vi "Z Aux Direct Move Smooth.vi"(0 "handle":u32, 1 "next1":sgl, 2 "next3":sgl, 5 "end1":sgl, 7 "end2":sgl, 9 "end3":sgl, 11 "error in (no error)":errorcluster caption="错误输入（无错误）", 12 "next2":sgl, 13 "radius":sgl) -> (4 "handle out":u32, 6 "function return":i32, 15 "error out":errorcluster caption="错误输出")   [LabVIEW 2015, in "zauxdll.lvlib"]
doc: "int32 __stdcall ZAux_Direct_MoveSmooth(ZMC_HANDLE handle, float end1, float end2, float end3, float next1, float next2, float next3, float radius);"
uses:
  zauxdll.lvlib
  zauxdll.dll
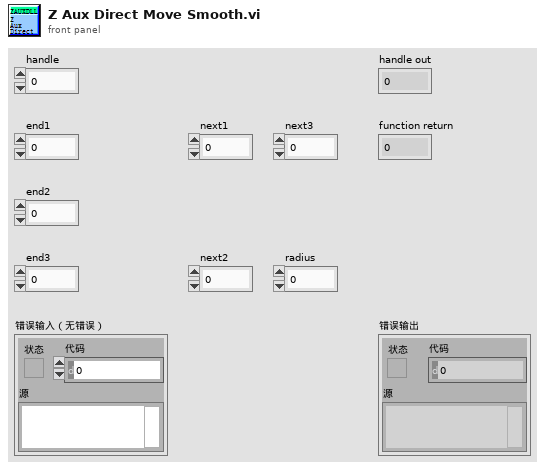
[diagram p1: front panel]
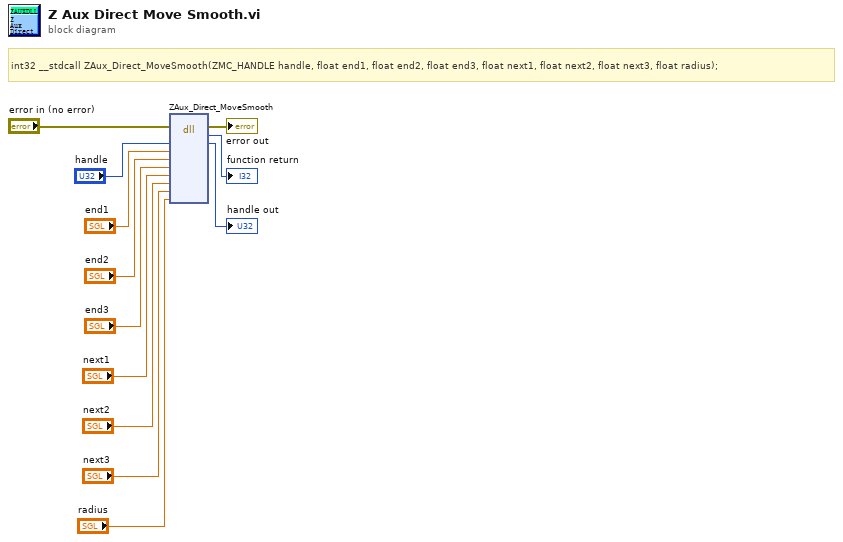
[diagram p0: block diagram]
diagram:
  # "int32 __stdcall ZAux_Direct_MoveSmooth(ZMC_HANDLE handle, float end1, float end2, float end3, float next1, float next2, float next3, float radius);"
  n1 = dll-call lib="C:/Users/VIC/Desktop/GOGORO_Oringnal - Panasonic/system/LLB/zmotion/zaux/zauxdll.*" fn="ZAux_Direct_MoveSmooth"(error in="error in (no error)", "handle"="handle", "end1"="end1", "end2"="end2", "end3"="end3", "next1"="next1", "next2"="next2", "next3"="next3", "radius"="radius") -> (error out=→"error out":errorcluster, →"function return":i32, "handle"=→"handle out":u32)  [unwired: 9 in, 1 out]
